vi "Read Section.vi"(8 "error in (no error)":errorcluster, 11 "Analyze Parameter Base in":refnum<class "Analyze Parameter Base.lvclass">) -> (0 "error out":errorcluster, 2 "Section":string="Parameters", 3 "Analyze Parameter Base out":refnum<class "Analyze Parameter Base.lvclass">)   [LabVIEW 2020, in "Analyze Parameter Base.lvclass"]
uses:
  Analyze Parameter Base.lvclass
  Analyze Parameter Base.lvclass/Analyze Parameter Base.ctl
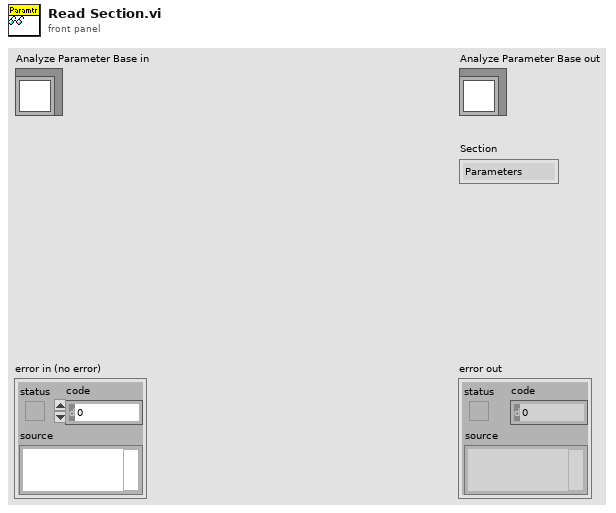
[diagram p1: front panel]
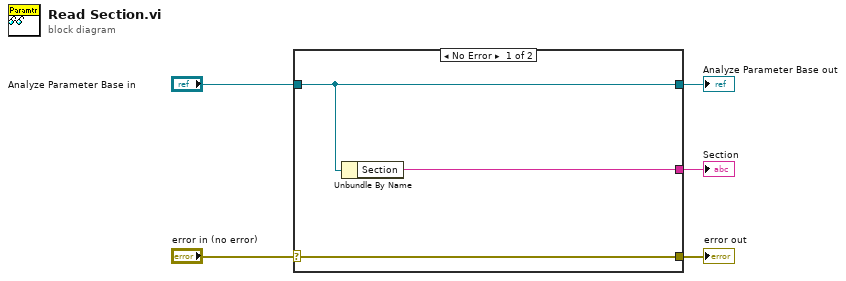
[diagram p0: block diagram]
diagram:
  n1 = case shown="No Error" "error in (no error)" {
    selector: "error in (no error)" -> [w8 w9]
    tunnel: [w8 w9] -> w4
    tunnel: [w7 w10] -> w2
    tunnel: "Analyze Parameter Base in" -> [w7 w10]
    tunnel: [w6 _] -> w1
    frame No Error {
      n2 = Unbundle By Name(w7) -> ("Section"=w6:string)
    }
    frame Error {
    }
  }
  "error out" <- w4
  "Analyze Parameter Base out" <- w2
  "Section" <- w1
